vi "Initail seq in.vi"() -> (0 "INI seq in":string[][](array[string])=[["0", "Top", "Top", "Top", "Top", "Top", "Top", "Top", "Top", "Top", "Top", "Top", "Top", "Top", "Top", "Top", "Top", "Top", "Top", "Top", "Top", "Top", "Top"], ["1", "Bottom", "Bottom", "Bottom", "Bottom", "Bottom", "Bottom", "Bottom", "Bottom", "Bottom", "Bottom", "Bottom", "Bottom", "Bottom", "Bottom", "Bottom", "Bottom", "Bottom", "Bottom", "Bottom", "Bottom", "Bottom", "Bottom"]])   [LabVIEW 2019]
panel:
  in  "list":i32[](listbox)
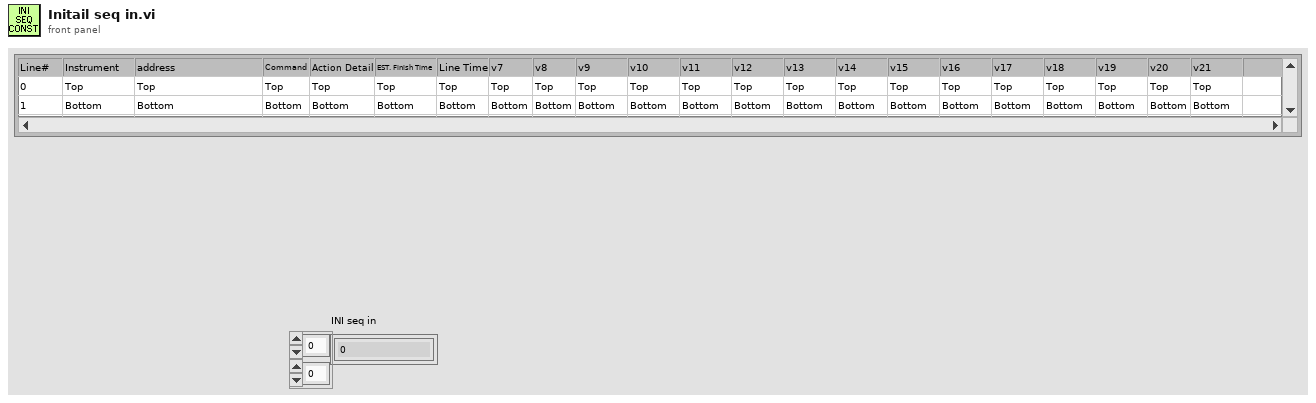
[diagram p1: front panel]
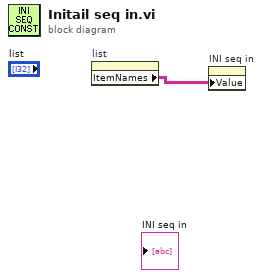
[diagram p0: block diagram]
diagram:
  n1 = property on="list" class="MCListbox (strict)"() -> ("ItemNames"=w1:string[][])  [unwired: 2 in, 2 out]
  n2 = property on="INI seq in" class="Arr (strict)"("Value"=w1) -> ()  [unwired: 2 in, 2 out]
